vi "Tag Names.vi"(11 "State In":T1={"State"=enum."Idle", "Start Time"=timestamp(0 s since 1904-01-01), "Configuration"={"Cycle Period"=0.0, "Ismatech"={"VISA resource name"="", "Simulated?"=FALSE, "Pump Number"=1.0, "Reverse?"=FALSE}, "Masterflex"={"VISA resource name"="", "Simulated?"=FALSE, "Pump Number"=1.0, "Reverse?"=FALSE}, "Manual Entry"=0.0, "VICI Settings"={"VISA resource name"="", "Simulated?"=FALSE, "Pump Letter"="", "Reverse?"=FALSE}, "Output Device"=enum."VICI", "Tacmina Settings"={"Analog DAQ Task"="", "Digital DAQ Task"=""}, "KNF SIMDOS Settings"={"VISA resource name"="", "Simulated?"=TRUE}, "ASIA Pump C"={"ASIA Pump #"=0, "channel"=0, "Simulated"=FALSE}, "FLOM Settings"={"VISA resource name"="", "Simulated?"=TRUE, "Pump Number"=0.0}, "Pump Calibration File"=path "", "Calibration Slope"=0.0, "Calibration Y Intercept"=0.0, "Pump Cal Enum"=0, "SSI PR Settings"={"VISA resource name"="", "Simulated?"=FALSE}}, "Current Time"=timestamp(0 s since 1904-01-01), "First Iteration"=FALSE, "Data"={"Pump Speed"=0.0, "Pump Pressure"=0.0, "Pump Flow"=0.0}, "Process Name"="", "Pump On?"=enum."Off", "Output Error"=FALSE, "Log Started"=FALSE, "Overpressure Alarming"=FALSE} {"Configuration"."ASIA Pump C"."channel" min=0 max=1 step=1; "Configuration"."Masterflex"."Pump Number" min=1.0 max=20.0 step=1.0; "Configuration"."Ismatech"."Pump Number" min=1.0 max=20.0 step=1.0}) -> (3 "Pump Module Tag Names":T13, 4 "All Boolean Tags":string[](array[string]), 5 "All  Numeric Tags":string[](array[string]))   [LabVIEW 2018, in "Pump Module.lvlib" / "Pump Module Engine.lvlib"]
uses:
  Pump Module Engine.lvlib
  Pump Module Tag Names Cluster.ctl
  State Cluster.ctl
  State Enum.ctl
  Pump Module Settings Cluster.ctl
  Ismatec ISM 831C/Controls/Ismatech Settings Cluster.ctl
  Masterflex 7550-30/Controls/Settings Cluster.ctl
  VICI M50 Party Mode/Settings Cluster.ctl
  Measure Instrument/PID 2 Output Enum.ctl
  Tacmina QI/Tacmina QI DAQ Setting.ctl
  KNF Pump/Settings Cluster plus SIMDOS.ctl
  ASIA Pump/Pump Settings.ctl
  FLOM Pump/Settings Cluster.ctl
  SSI PR Class/SSI PR Settings Cluster.ctl
  Pump Module.lvlib
  Ismatec ISM 831C/Ismatec ISM 831C.lvlib
  Masterflex 7550-30/Masterflex 7550-30.lvlib
  VICI M50 Party Mode/VICI M6 M50 Party Mode.lvlib
  Tacmina QI/Tacmina QI.lvlib
  KNF Pump/KNF SIMDOS.lvlib
  ASIA Pump.lvlib
  FLOM Pump/FLOM Pump.lvlib
  SSI PR Class/SSI PR Pump.lvlib
panel:
  # "Output Instruments"
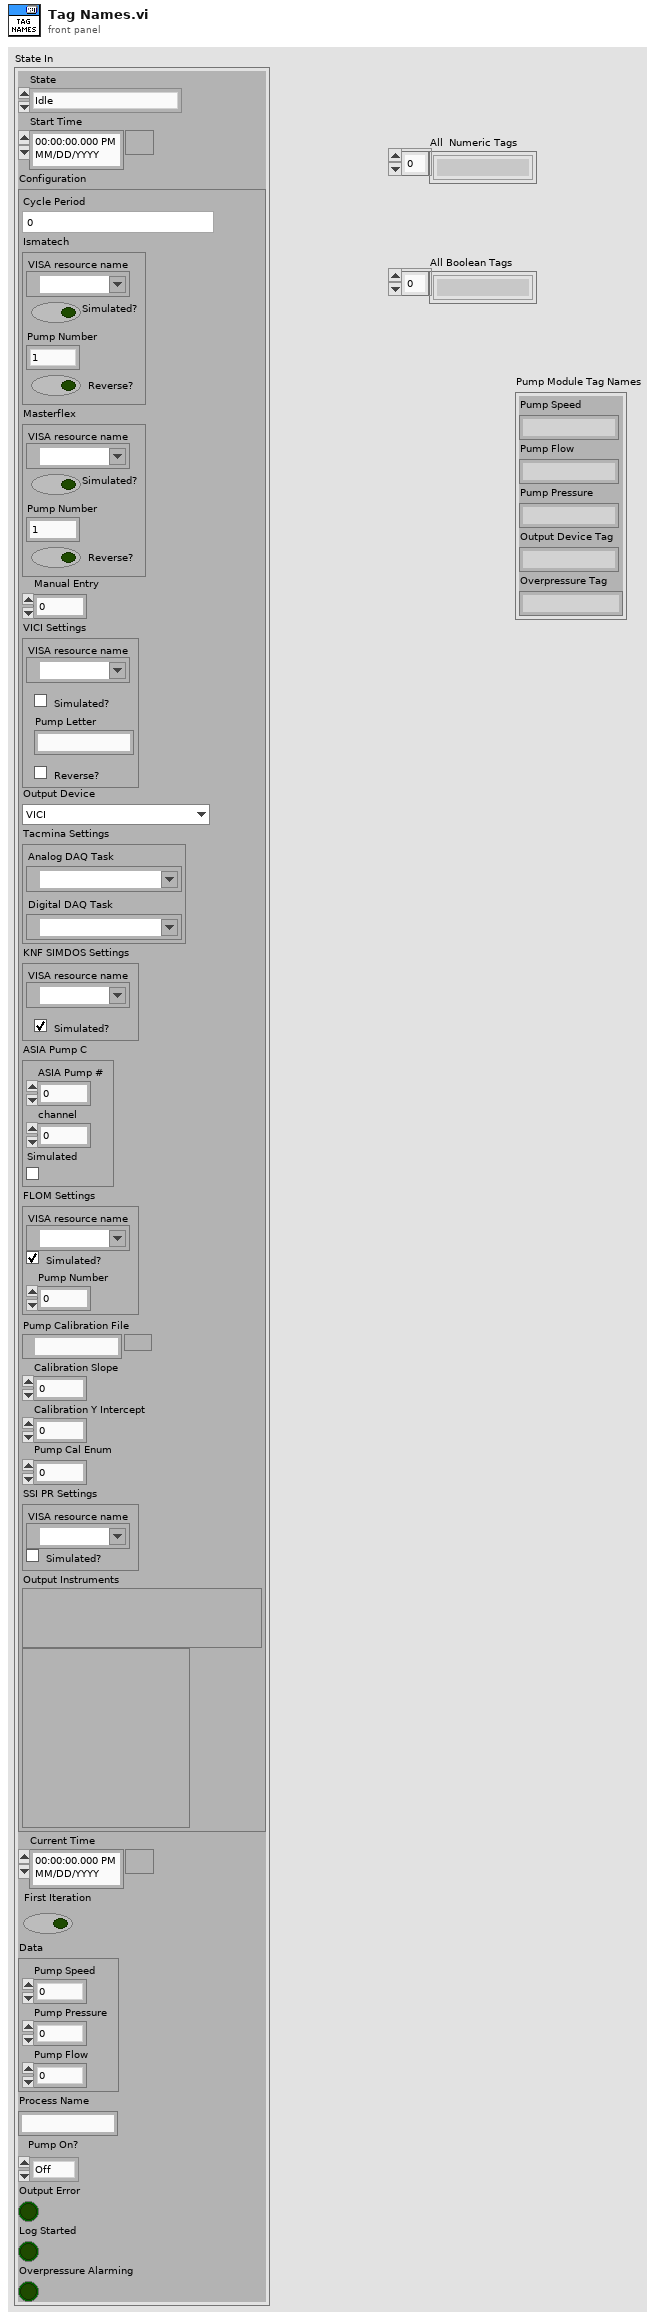
[diagram p1: front panel]
types:
  T1 = typedef "Pump Module.lvlib/Pump Module Engine.lvlib/State Cluster.ctl" = cluster{"State":T2, "Start Time":timestamp, "Configuration":T3, "Current Time":timestamp, "First Iteration":bool, "Data":cluster{"Pump Speed":dbl, "Pump Pressure":dbl, "Pump Flow":dbl}, "Process Name":string, "Pump On?":enum16{"Off", "On", "Not Initialized"}, "Output Error":bool, "Log Started":bool, "Overpressure Alarming":bool}
  T2 = typedef "Pump Module.lvlib/Pump Module Engine.lvlib/State Enum.ctl" = enum16{"Measuring", "Idle", "Paused"}
  T3 = typedef "Pump Module.lvlib/Pump Module Settings Cluster.ctl" = cluster{"Cycle Period":dbl, "Ismatech":T4, "Masterflex":T5, "Manual Entry":dbl, "VICI Settings":T6, "Output Device":T7, "Tacmina Settings":T8, "KNF SIMDOS Settings":T9, "ASIA Pump C":T10, "FLOM Settings":T11, "Pump Calibration File":path, "Calibration Slope":dbl, "Calibration Y Intercept":dbl, "Pump Cal Enum":u16, "SSI PR Settings":T12}
  T4 = typedef "Ismatec ISM 831C.lvlib/Ismatech Settings Cluster.ctl" = cluster{"VISA resource name":refnum<visa-resource-name>, "Simulated?":bool, "Pump Number":dbl, "Reverse?":bool}
  T5 = typedef "Masterflex 7550-30.lvlib/Settings Cluster.ctl" = cluster{"VISA resource name":refnum<visa-resource-name>, "Simulated?":bool, "Pump Number":dbl, "Reverse?":bool}
  T6 = typedef "VICI M6 M50 Party Mode.lvlib/Settings Cluster.ctl" = cluster{"VISA resource name":refnum<visa-resource-name>, "Simulated?":bool, "Pump Letter":string, "Reverse?":bool}
  T7 = typedef "PID 2 Output Enum.ctl" = enum16{"Default", "Ismatec ISM 831C", "Masterflex 7550-30", "VICI", "Tacmina QI", "KNF SIMDOS", "ASIA Type C", "FLOM UI-22-11", "SSI PR"}
  T8 = typedef "Tacmina QI.lvlib/Tacmina QI DAQ Setting.ctl" = cluster{"Analog DAQ Task":refnum<k21>, "Digital DAQ Task":refnum<k21>}
  T9 = typedef "KNF SIMDOS.lvlib/Settings Cluster plus SIMDOS.ctl" = cluster{"VISA resource name":refnum<visa-resource-name>, "Simulated?":bool}
  T10 = typedef "ASIA Pump.lvlib/Pump Settings.ctl" = cluster{"ASIA Pump #":i32, "channel":i32, "Simulated":bool}
  T11 = typedef "FLOM Pump.lvlib/Settings Cluster.ctl" = cluster{"VISA resource name":refnum<visa-resource-name>, "Simulated?":bool, "Pump Number":dbl}
  T12 = typedef "SSI PR Pump.lvlib/SSI PR Settings Cluster.ctl" = cluster{"VISA resource name":refnum<visa-resource-name>, "Simulated?":bool}
  T13 = typedef "Pump Module.lvlib/Pump Module Tag Names Cluster.ctl" = cluster{"Pump Speed":string, "Pump Flow":string, "Pump Pressure":string, "Output Device Tag":string, "Overpressure Tag":string}
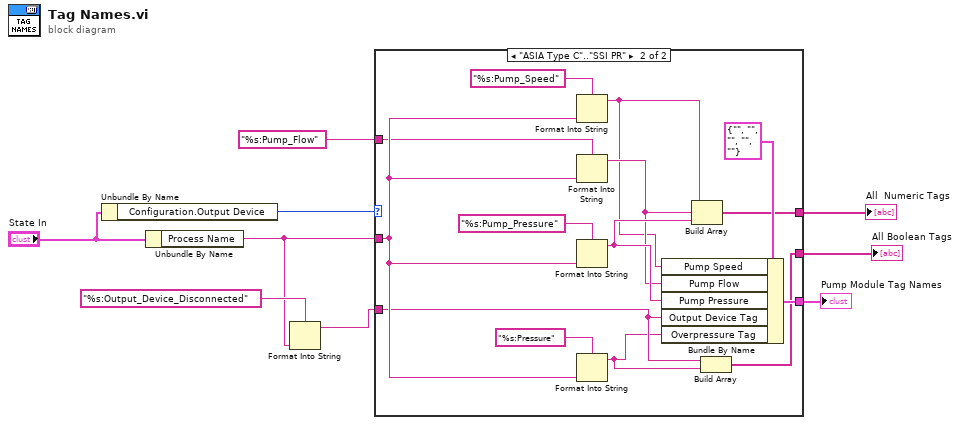
[diagram p0: block diagram]
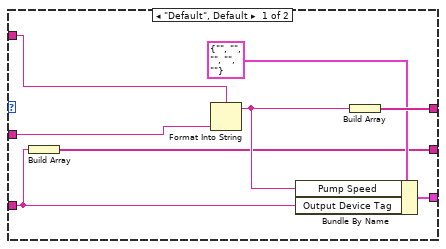
[diagram p2: hidden frame]
diagram:
  n1 = Unbundle By Name("State In") -> ("Configuration.Output Device"=w8:T7)
  n2 = Unbundle By Name("State In") -> ("Process Name"=w4:string)
  n3 = Format Into String(format string="%s:Output_Device_Disconnected", w4) -> (resulting string=w2:string)  [unwired: 2 in, 1 out]
  n4 = case shown="\"ASIA Type C\"..\"SSI PR\"" w8 {
    tunnel: w4 -> [w16 w22]
    tunnel: w2 -> [w12 w21]
    tunnel: [w17 w26] -> w6
    tunnel: [w14 w25] -> w7
    tunnel: [w11 w20] -> w3
    tunnel: "%s:Pump_Flow" ("format string") -> [w10 w18]
    frame "Default", Default {
      n5 = Build Array(w12) -> (w11:string[])
      n6 = Format Into String(format string=w10, w16) -> (resulting string=w15:string)  [unwired: 2 in, 1 out]
      n7 = Bundle By Name(cluster=T13 {"Pump Speed"="", "Pump Flow"="", "Pump Pressure"="", "Output Device Tag"="", "Overpressure Tag"=""} ("Feed Module Tag Names"), "Pump Speed"=w15, "Output Device Tag"=w12) -> (w14:T13)
      n8 = Build Array(w15) -> (w17:string[])
    }
    frame "ASIA Type C".."SSI PR" {
      n9 = Format Into String(format string="%s:Pump_Speed", w22) -> (resulting string=w24:string)  [unwired: 2 in, 1 out]
      n10 = Format Into String(format string=w18, w22) -> (resulting string=w30:string)  [unwired: 2 in, 1 out]
      n11 = Format Into String(format string="%s:Pump_Pressure", w22) -> (resulting string=w31:string)  [unwired: 2 in, 1 out]
      n12 = Format Into String(format string="%s:Pressure", w22) -> (resulting string=w19:string)  [unwired: 2 in, 1 out]
      n13 = Bundle By Name(cluster=T13 {"Pump Speed"="", "Pump Flow"="", "Pump Pressure"="", "Output Device Tag"="", "Overpressure Tag"=""} ("Feed Module Tag Names"), "Pump Speed"=w24, "Pump Flow"=w30, "Pump Pressure"=w31, "Output Device Tag"=w21, "Overpressure Tag"=w19) -> (w25:T13)
      n14 = Build Array(w24, w30, w31) -> (w26:string[])
      n15 = Build Array(w21, w19) -> (w20:string[])
    }
  }
  "Pump Module Tag Names" <- w7
  "All Boolean Tags" <- w3
  "All  Numeric Tags" <- w6
